vi "Open System Definition.vi"(8 "error in (no error)":errorcluster, 11 "System Definition File":path) -> (0 "error out":errorcluster, 1 "Target Refnum":refnum<k24>, 2 "Root Refnum":refnum<k24>, 3 "System Definition Refnum":refnum<k24>)   [LabVIEW 2019]
uses:
  NationalInstruments.VeriStand.SystemDefinitionAPI
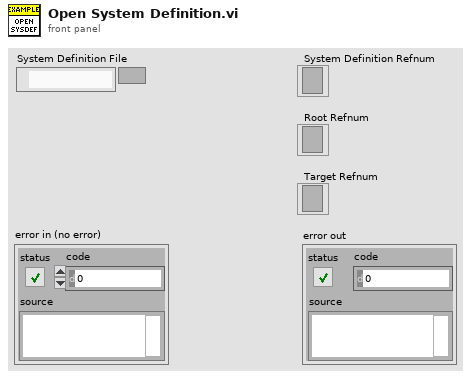
[diagram p1: front panel]
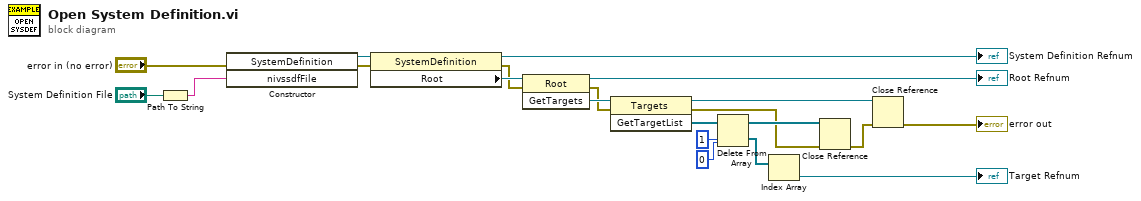
[diagram p0: block diagram]
diagram:
  n1 = Path To String(path="System Definition File") -> (string=w1:string)
  n2 = constructor class="SystemDefinition"(error in="error in (no error)", "nivssdfFile"=w1) -> (reference out=w5:refnum<k24>, error out=w4:errorcluster)  [unwired: 2 in, 2 out]
  n3 = property class="SystemDefinition"(reference=w5, error in=w4) -> (reference out=→"System Definition Refnum":refnum<k24>, error out=w6:errorcluster, "Root"=w7:refnum<k24>)
  n4 = invoke class="Root" method="GetTargets"(reference=w7, error in=w6) -> (reference out=→"Root Refnum":refnum<k24>, error out=w8:errorcluster, "GetTargets"=w9:refnum<k24>)  [unwired: 1 in]
  n5 = invoke class="Targets" method="GetTargetList"(reference=w9, error in=w8) -> (reference out=w16:refnum<k24>, error out=w13:errorcluster, "GetTargetList"=w10:refnum<k24>[])  [unwired: 1 in]
  n6 = Delete From Array(array=w10, length=1, index=0) -> (deleted portion=w17:refnum<k24>[], array with subset deleted=w14:refnum<k24>[])
  n7 = Index Array(array=w17) -> (element=→"Target Refnum":refnum<k24>)  [unwired: 1 in]
  n8 = Close Reference(reference=w14, error in (no error)=w13) -> (error out=w15:errorcluster)
  n9 = Close Reference(reference=w16, error in (no error)=w15) -> (error out=→"error out":errorcluster)
